vi "Remove.vi"() -> ()   [LabVIEW 2024, in "VarCircularBuffer.Tests.Units.lvlib"]
uses:
  VarCircularBuffer.Tests.Units.lvlib
  VarCircularBuffer.lvclass/VarCircularBuffer.ctl
  Flush.vi/9e5e380d-a9b6-4c49-a1d6-4829efd6953e.vi
  Flush.vi/9e5e380d-a9b6-4c49-a1d6-4829efd6953e.vi/83cdeaba-e1ff-493a-b62c-1f93efcfb5e6.vi
  <vilib>/addons/_JKI Toolkits/Caraya/classes/Assert/Assert True.vi
  <vilib>/addons/_JKI Toolkits/Caraya/classes/Assert/Assert False.vi
  <vilib>/addons/_JKI Toolkits/Caraya/classes/Assert/Assert.lvclass
  <vilib>/addons/_JKI Toolkits/Caraya/classes/Test/Test.lvclass
  VarCircularBuffer.lvclass
panel:
  in  "expected":variant[](array[variant])=[variant(i32 2), variant(i32 3), variant(i32 4), variant(i32 5), variant(i32 6), variant(i32 7), variant(i32 8), variant(i32 9), variant(i32 10)]
  out "element":variant=variant(i32 0)
  out "Flushed Buffer":variant[](array[variant])
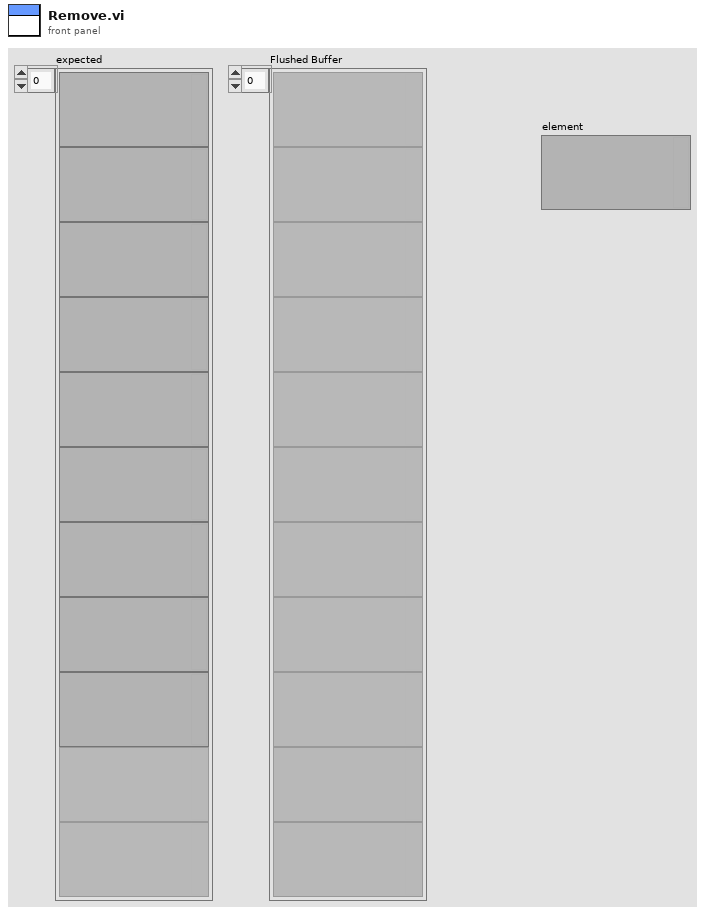
[diagram p1: front panel]
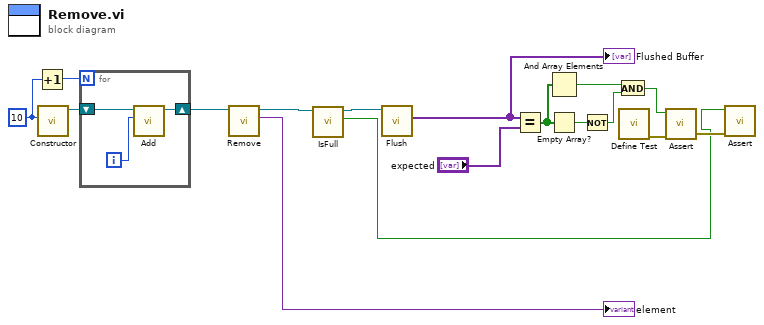
[diagram p0: block diagram]
diagram:
  w15 = u32 10 ("Capacity")
  n1 = Increment(x=w15) -> (x+1=w16:u32)
  n2 = call "Constructor.vi"("Capacity"=w15) -> ("TypedCircularBuffer out"=w17:refnum<class "VarCircularBuffer.lvclass">)  [unwired: 10 in]
  n3 = for {
    N: w16 -> [_]
    shift-right: [w19] -> w7
    shift-left: w17 -> [w20]
    i -> [w18]
    n4 = call "Add.vi"("Element"=w18, "TypedCircularBuffer in"=w20) -> ("TypedCircularBuffer out"=w19:refnum<class "VarCircularBuffer.lvclass">)  [unwired: 7 in, 2 out]
  }
  n5 = call "Remove.vi"("TypedCircularBuffer in"=w7) -> ("element"=→"element":variant, "TypedCircularBuffer out"=w5:refnum<class "VarCircularBuffer.lvclass">)  [unwired: 8 in, 1 out]
  n6 = call "IsFull.vi"("TypedCircularBuffer in"=w5) -> ("Full?"=w2:bool, "TypedCircularBuffer out"=w4:refnum<class "VarCircularBuffer.lvclass">)  [unwired: 9 in]
  n7 = call "Flush.vi"("TypedCircularBuffer in"=w4) -> ("Flushed Buffer"=w8:variant[])  [unwired: 9 in, 1 out]
  "Flushed Buffer" <- w8
  n8 = Equal?(x=w8, y="expected") -> (x = y?=w11:bool[])
  n9 = And Array Elements(Boolean array=w11) -> (logical AND=w14:bool)
  n10 = Empty Array?(array=w11) -> (empty?=w13:bool)
  n11 = Not(x=w13) -> (.not. x?=w12:bool)
  n12 = And(x=w14, y=w12) -> (x .and. y?=w10:bool)
  n13 = call <vilib>:"Define Test.vi"() -> ("error out"=w9:errorcluster)  [unwired: 10 in, 1 out]
  n14 = call-poly <vilib>:"Assert.vi"("error in (no error)"=w9, "True?"=w10) -> ("error out"=w3:errorcluster)  [unwired: 8 in, 1 out]
  n15 = call-poly <vilib>:"Assert.vi"("error in (no error)"=w3, "False?"=w2) -> ()  [unwired: 8 in, 2 out]
